vi "Destroy.vi"(8 "error in (no error)":errorcluster) -> (0 "error out":errorcluster)   [LabVIEW 2016, in "Global_logger.lvlib"]
uses:
  Global_logger.lvlib
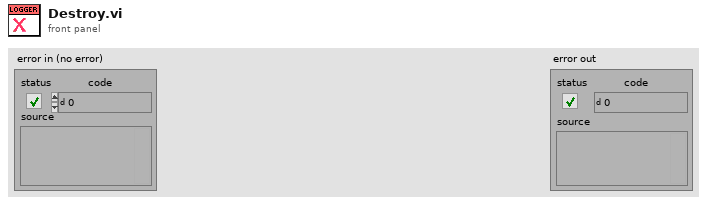
[diagram p1: front panel]
types:
  T1 = typedef "Global_logger.lvlib/Options.ctl" = cluster{"filesize (bytes)":u32, "logs max age (days) ":u16, "write per N messages":u16}
  T2 = typedef "Global_logger.lvlib/Levels.ctl" = enum16{"ALL", "TRACE", "DEBUG", "INFO", "WARN", "ERROR", "FATAL", "OFF"}
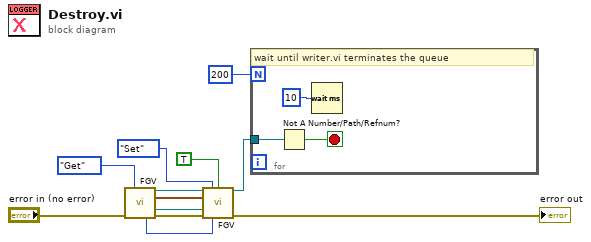
[diagram p0: block diagram]
diagram:
  n1 = call "FGV.vi"("Action"=enum16{"Get", "Set"}."Get", "error in (no error)"="error in (no error)") -> ("queue out"=w11:refnum<queue>, "Options out"=w8:T1, "Root Logging Path out"=w7:path, "Level out"=w5:T2, "error out"=w6:errorcluster)  [unwired: 8 in, 1 out]
  n2 = call "FGV.vi"("queue in"=w11, "Action"=enum16{"Get", "Set"}."Set", "Destroy Logger in"=TRUE, "Options in"=w8, "Root Logging Path in"=w7, "error in (no error)"=w6, "Level in"=w5) -> ("queue out"=w2:refnum<queue>, "error out"=→"error out":errorcluster)  [unwired: 3 in, 4 out]
  n3 = for {
    N: 200 -> [_]
    tunnel: w2 -> [w14]
    stop <- w13 stop-if-true
    # "wait until writer.vi terminates the queue"
    n4 = Not A Number/Path/Refnum?(number/path/refnum=w14) -> (NaN/Path/Refnum?=w13:bool)
    n5 = Wait (ms)(milliseconds to wait=u32 10) -> ()  [unwired: 1 out]
  }
